vi "Create Graph Plot Arrays.vi"(8 "error in":errorcluster, 10 "InverterWaveforms":T1) -> (0 "error out":errorcluster, 1 "DUT1 60 Hz V and I":waveform(dbl)[](array[waveform]), 2 "Iouts 60Hz":waveform(dbl)[](array[waveform]), 3 "DUT4 60 Hz V and I":waveform(dbl)[](array[waveform]), 4 "DUT2 60 Hz V and I":waveform(dbl)[](array[waveform]), 5 "Iout ripples":waveform(dbl)[](array[waveform]), 6 "DUT3 60 Hz V and I":waveform(dbl)[](array[waveform]), 7 "Iin ripples":waveform(dbl)[](array[waveform]))   [LabVIEW 2019, in "Main.lvclass"]
doc: "Developed by Kevin Thompson\nkevin@thompsonengineering.net\n\nCopyright 2020\nThompson Engineering, LLC"
uses:
  Main.lvclass
  Common/DataTypes/InverterWaveforms--cluster.ctl
  Common/DataTypes/ChannelWaveforms--cluster.ctl
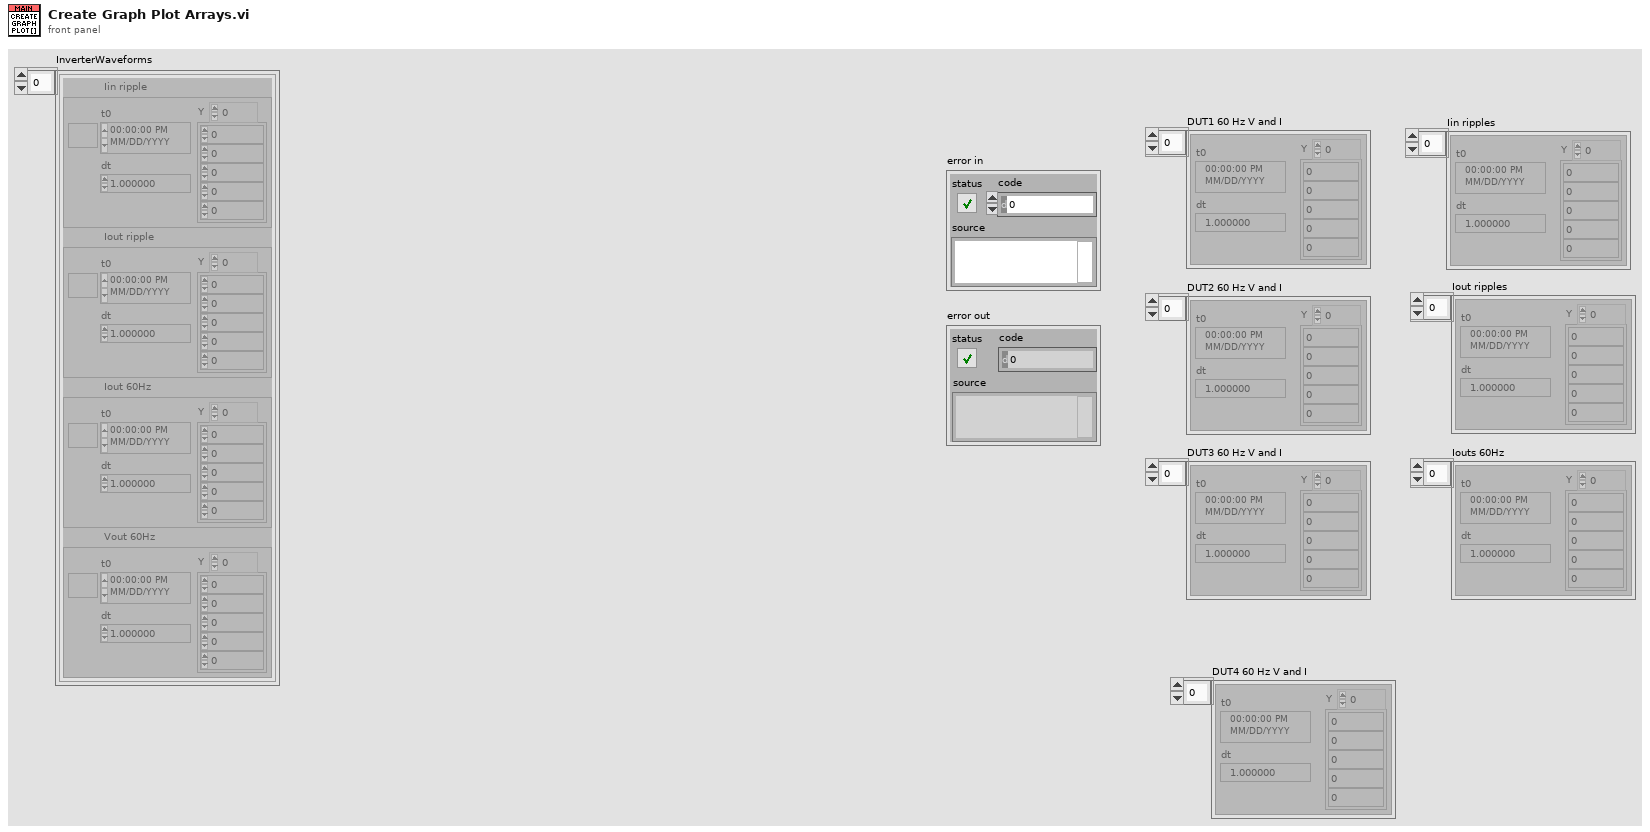
[diagram p1: front panel]
types:
  T1 = typedef "InverterWaveforms--cluster.ctl" = T2[]
  T2 = typedef "ChannelWaveforms--cluster.ctl" = cluster{"Iin ripple ":waveform(dbl), "Iout ripple ":waveform(dbl), "Iout 60Hz":waveform(dbl), "Vout 60Hz":waveform(dbl)}
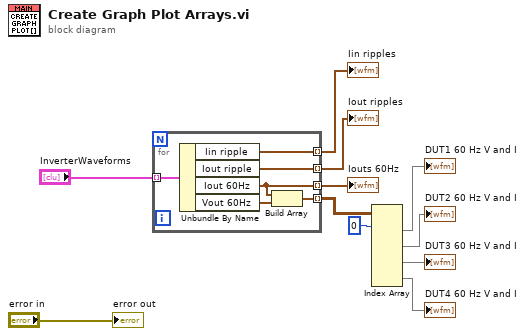
[diagram p0: block diagram]
diagram:
  n1 = for {
    tunnel: "InverterWaveforms" -> [w17] mode=indexing
    tunnel: [w16] -> w9 mode=indexing
    tunnel: [w15] -> w8 mode=indexing
    tunnel: [w12] -> w7 mode=indexing
    tunnel: [w13] -> w6 mode=indexing
    n2 = Unbundle By Name(w17) -> ("Iin ripple"=w16:waveform(dbl), "Iout ripple"=w15:waveform(dbl), "Iout 60Hz"=w12:waveform(dbl), "Vout 60Hz"=w14:waveform(dbl))
    n3 = Build Array(w12, w14) -> (w13:waveform(dbl)[])
  }
  "Iin ripples" <- w9
  "Iout ripples" <- w8
  "Iouts 60Hz" <- w7
  n4 = Index Array(array=w6, index (row) #1=0 ("disabled index (col)")) -> (element #1=→"DUT1 60 Hz V and I":waveform(dbl)[], element #2=→"DUT2 60 Hz V and I":waveform(dbl)[], element #3=→"DUT3 60 Hz V and I":waveform(dbl)[], element #4=→"DUT4 60 Hz V and I":waveform(dbl)[])  [unwired: 7 in]
  "error out" <- "error in"
